vi "gain ranging test FSM.vi"(0 "gain ranging.start sequence":bool, 5 "gain ranging.dwell time (cycles)":u32=4800, 7 "gain ranging.gain setting list":T5, 9 "gain ranging.manual request":T3) -> (4 "gain ranging.gain setting":fxp<+/-,16,12>, 6 "gain ranging.TX1/RX1 Port Value":T1=enum."TX1/RX2", 8 "gain ranging.start of sequence":bool, 10 "gain ranging.gain setting valid":bool)   [LabVIEW 2019]
uses:
  Host/SubVIs/Low-level/TypeDefs/Gain Setting.ctl
  <instrlib>/niMmWave/ni3620/Config/v1/FPGA/Public/Typedefs/TX1 RX1 Port.ctl
  <vilib>/rvi/DataTransferAndStorage/Container/Common/niFpgaContainerGetUniqueNameForEmu.vi
  <vilib>/rvi/DataTransferAndStorage/Container/Common/niFpgaContainerSetEmuInfo.vi
  <vilib>/rvi/eio/common/nirviEmuReportErrorAndStop.vi
  <vilib>/rvi/DataTransferAndStorage/Container/Common/niFpgaContainerExecOnDevCompGetState.vi
  <vilib>/rvi/Emulation/niFpgaEmulationIsFPGAContextNoSignature.vi
  <vilib>/rvi/Emulation/niFpgaProcessEmulError.vi
  <vilib>/rvi/Emulation/niFpgaSctlEmulationGetInTimedLoop.vi
  <vilib>/rvi/errors/nirviReportUnexpectedCaseInternalError (U32).vi
  <vilib>/rvi/Memory/Memory_Emulation/niFpgaMemoryEmulationCacheClearOnFirstRun.vi
  <vilib>/rvi/Memory/Memory_Emulation/nirvimemoryEmulationManagerCache_MakeExclusive.vi
  <vilib>/rvi/Memory/Memory_Emulation/niFpgaMemoryEmulationValidateCache.vi
  <vilib>/rvi/Memory/Memory_Emulation/nirvimemoryEmulationManagerCache_InsertValue.vi
  <vilib>/Utility/error.llb/Clear Errors.vi
  <vilib>/rvi/Memory/Memory_Emulation/nirvimemoryEmulationManagerCache_ReleaseExclusive.vi
  <vilib>/rvi/Memory/Memory_Emulation/nirvimemoryEmulationManagerCache_GetValue.vi
  <vilib>/rvi/Memory/Memory_Emulation/nirvimemoryEmulationManagerCache_SetValue.vi
  <vilib>/rvi/Emulation/niFpgaSctlEmulationResourceMgr.vi
  <instrlib>/_niInstr/Basic Elements/v1/FPGA/Private/Count Up U16.vi
  <instrlib>/_niInstr/Basic Elements/v1/FPGA/Private/Count Down U32.vi
  <vilib>/rvi/LocalResourceManager/LocalResourceManager.xnode
  <vilib>/rvi/DataTransferAndStorage/Container/XNode/niFpgaContainer.xnode
  <vilib>/rvi/Memory/Memory_Emulation/niFpgaMemoryEmulationRefIn.vi
  <instrlib>/_niInstr/Basic Elements/v1/FPGA/niInstr Basic Elements v1 FPGA.lvlib
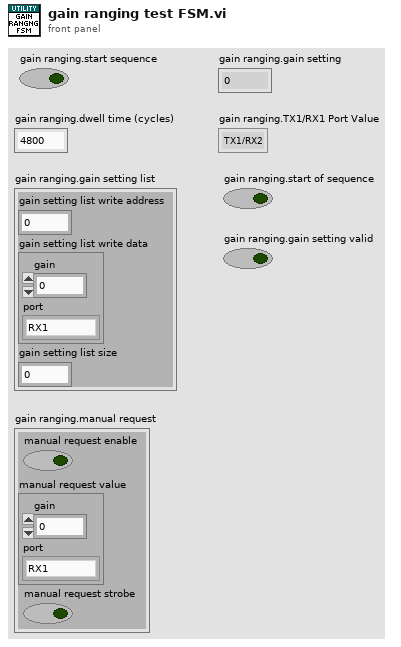
[diagram p1: front panel]
types:
  T1 = typedef "TX1 RX1 Port.ctl" = enum8{"RX1", "TX1/RX2"}
  T2 = typedef "Gain Setting.ctl" = cluster{"gain":fxp<+/-,16,12>, "port":T1}
  T3 = cluster{"manual request enable":bool, "manual request value":T2, "manual request strobe":bool}
  T4 = typedef "gain setting.ctl" = cluster{"gain":fxp<+/-,16,12>, "port":T1}
  T5 = cluster{"gain setting list write address":u32, "gain setting list write data":T4, "gain setting list size":u16}
  T6 = cluster{"gain":fxp<+/-,16,12>, "port":enum8{"RX1", "TX1/RX2"}}
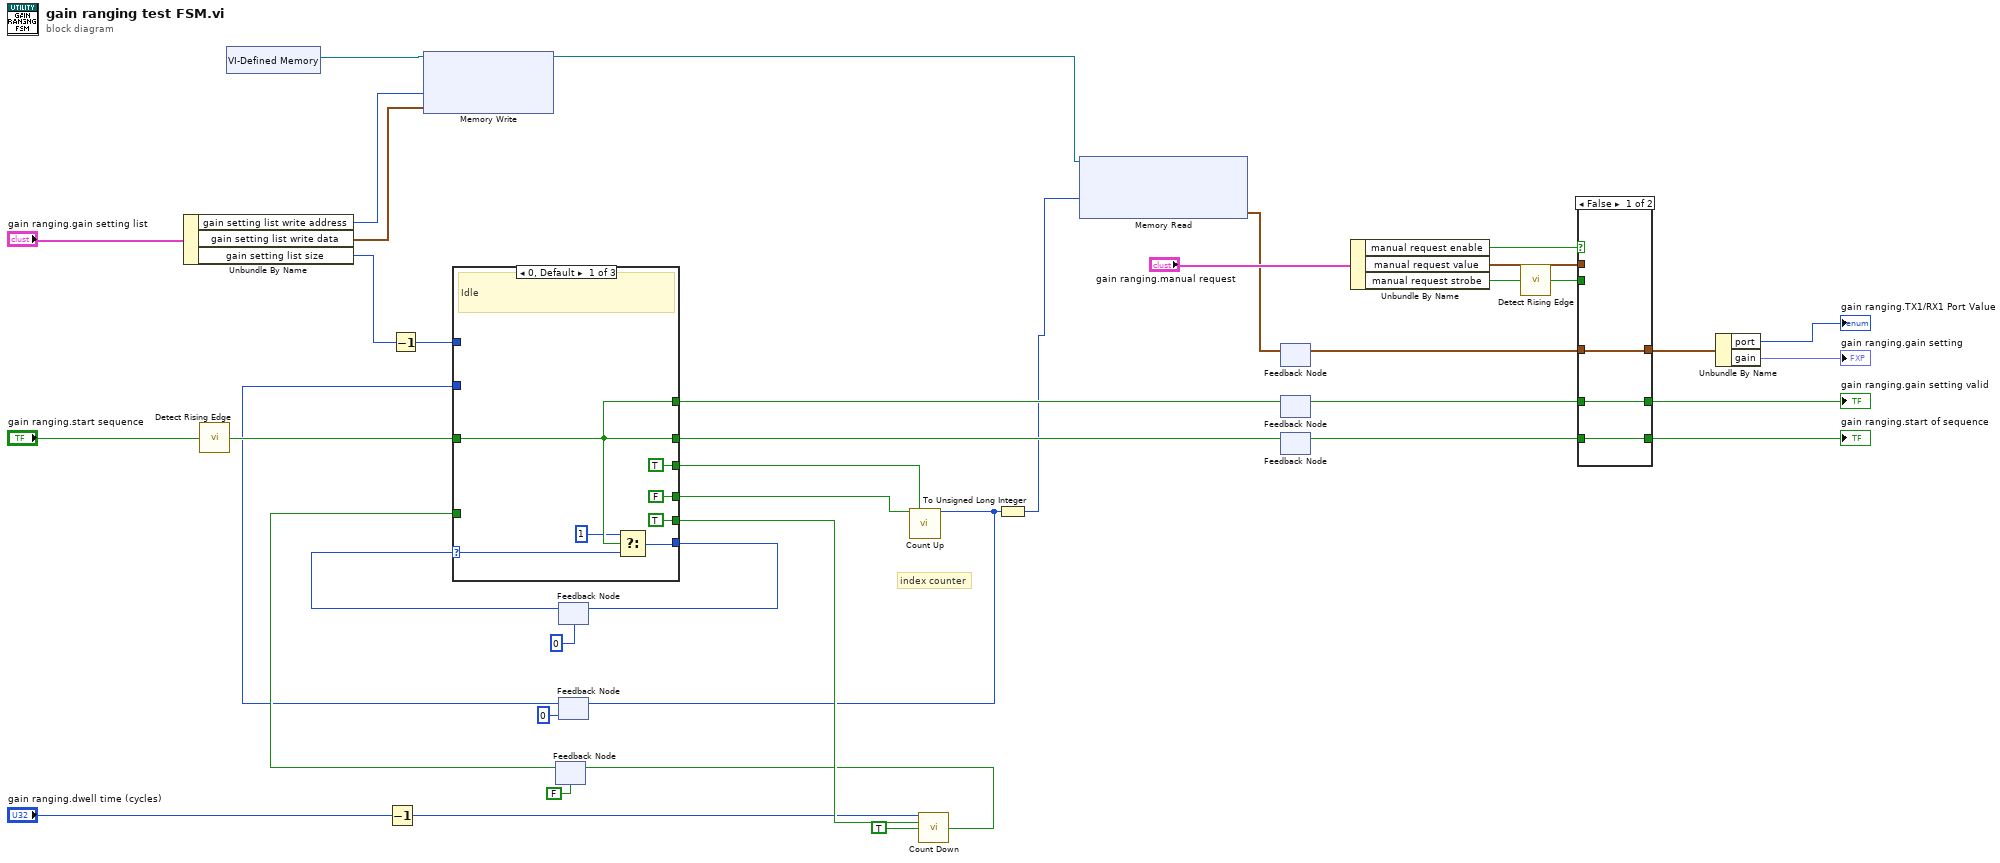
[diagram p0: block diagram]
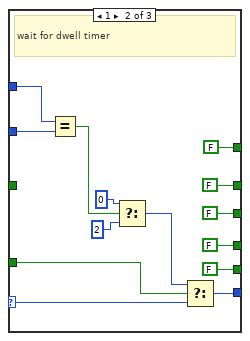
[diagram p2: hidden frame]
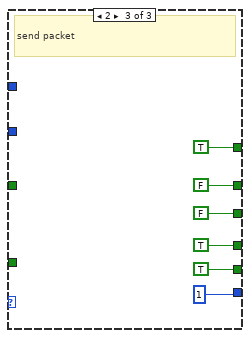
[diagram p3: hidden frame]
diagram:
  # "index counter"
  n1 = Unbundle By Name("gain ranging.gain setting list") -> ("gain setting list write address"=w5:u32, "gain setting list write data"=w4:T4, "gain setting list size"=w14:u16)
  n2 = call <instrlib>:"Detect Rising Edge.vi"("signal"="gain ranging.start sequence") -> ("edge detected"=w30:bool)  [unwired: 14 in]
  n3 = xnode "VI-Defined Memory"() -> ("Memory Out"=w6:refnum<k21>)
  n4 = Decrement(x="gain ranging.dwell time (cycles)") -> (x-1=w16:u32)
  n5 = Decrement(x=w14) -> (x-1=w19:u16)
  n6 = xnode "Memory Write"("Address"=w5, "Data"=w4, "Memory In"=w6) -> ("Memory Out"=w3:refnum<k21>)
  n7 = feedback #1(FALSE ("terminal count")) -> (w23:bool)
  n8 = feedback #2(u8 0) -> (w31:u8)
  n9 = feedback #3(u16 0) -> (w20:u16)
  n10 = case shown="0, Default" w31 {
    selector: w31 -> [w48 w60 _]
    tunnel: w30 -> [w45 _ _]
    tunnel: [w47 w61 u8 1 ("t")] -> w29
    tunnel: [w45 FALSE FALSE] -> w40
    tunnel: [TRUE ("edge detected") FALSE ("edge detected") TRUE ("edge detected")] -> w28
    tunnel: [TRUE ("edge detected") FALSE ("edge detected") FALSE ("edge detected")] -> w26
    tunnel: [FALSE ("edge detected") FALSE ("edge detected") TRUE ("edge detected")] -> w25
    tunnel: w23 -> [_ w59 _]
    tunnel: w20 -> [_ w52 _]
    tunnel: w19 -> [_ w53 _]
    tunnel: [w45 FALSE ("edge detected") TRUE ("edge detected")] -> w38
    frame 0, Default {
      # "Idle"
      n11 = Select(t=u8 1, s=w45, f=w48) -> (s? t:f=w47:u8)
    }
    frame 1 {
      # "wait for dwell timer"
      n12 = Equal?(x=w53, y=w52) -> (x = y?=w50:bool)
      n13 = Select(t=u8 0, s=w50, f=u8 2 ("t")) -> (s? t:f=w51:u8)
      n14 = Select(t=w51, s=w59, f=w60) -> (s? t:f=w61:u8)
    }
    frame 2 {
      # "send packet"
    }
  }
  n15 = feedback-in #2(w29) -> ()
  n16 = call-poly <instrlib>:"Count Up.vi"("increment"=w25, "reset"=w26) -> ("count out"=w18:u16)  [unwired: 13 in]
  n17 = feedback-in #3(w18) -> ()
  n18 = call-poly <instrlib>:"Count Down.vi"("count in"=w16, "load"=w28, "decrement"=TRUE) -> ("terminal count"=w24:bool)  [unwired: 11 in, 1 out]
  n19 = feedback-in #1(w24) -> ()
  n20 = To Unsigned Long Integer(number=w18) -> (unsigned 32bit integer=w2:u32)
  n21 = xnode "Memory Read"("Address"=w2, "Memory In"=w3) -> ("Data"=w1:T6)  [unwired: 1 out]
  n22 = feedback #4() -> (w37:T6)  [unwired: 1 in]
  n23 = feedback-in #4(w1) -> ()
  n24 = feedback #5() -> (w39:bool)  [unwired: 1 in]
  n25 = feedback-in #5(w38) -> ()
  n26 = feedback #6() -> (w41:bool)  [unwired: 1 in]
  n27 = feedback-in #6(w40) -> ()
  n28 = Unbundle By Name("gain ranging.manual request") -> ("manual request enable"=w12:bool, "manual request value"=w11:T2, "manual request strobe"=w10:bool)
  n29 = call <instrlib>:"Detect Rising Edge.vi"("signal"=w10) -> ("edge detected"=w33:bool)  [unwired: 14 in]
  n30 = case shown="False" w12 {
    tunnel: [w71 w73] -> w9
    tunnel: w37 -> [w71 _]
    tunnel: [w69 w72] -> w36
    tunnel: w11 -> [_ w73]
    tunnel: w33 -> [_ w72]
    tunnel: w41 -> [w70 _]
    tunnel: [w70 w72] -> w35
    tunnel: w39 -> [w69 _]
    frame False {
    }
    frame True {
    }
  }
  "gain ranging.gain setting valid" <- w36
  "gain ranging.start of sequence" <- w35
  n31 = Unbundle By Name(w9) -> ("port"=→"gain ranging.TX1/RX1 Port Value":T1, "gain"=→"gain ranging.gain setting":fxp<+/-,16,12>)
